vi "hmi_peg_leg.vi"(11 "UserData":T1) -> ()   [LabVIEW 2011]
uses:
  user_data.ctl
  user_buttons_dualaction.ctl
  user_buttons_360.ctl
  joe_johnson/peg_leg_state.ctl
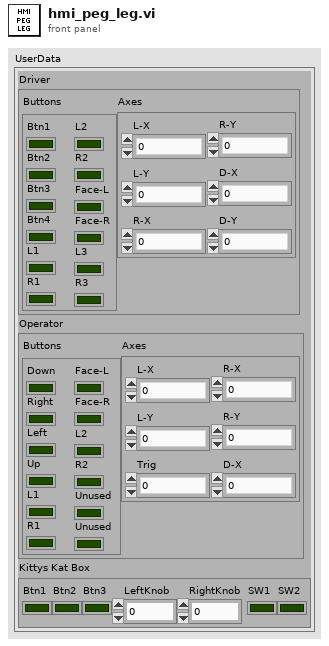
[diagram p1: front panel]
types:
  T1 = typedef "user_data.ctl" = cluster{"Driver":cluster{"Buttons":T2, "Axes":cluster{"L-X":dbl, "L-Y":dbl, "R-X":dbl, "R-Y":dbl, "D-X":dbl, "D-Y":dbl}}, "Operator":cluster{"Buttons":T3, "Axes":cluster{"L-X":dbl, "L-Y":dbl, "Trig":dbl, "R-X":dbl, "R-Y":dbl, "D-X":dbl}}, "Kittys Kat Box":cluster{"Btn1":bool, "Btn2":bool, "Btn3":bool, "LeftKnob":dbl, "RightKnob":dbl, "SW1":bool, "SW2":bool}}
  T2 = typedef "user_buttons_dualaction.ctl" = cluster{"Btn1":bool, "Btn2":bool, "Btn3":bool, "Btn4":bool, "L1":bool, "R1":bool, "L2":bool, "R2":bool, "Face-L":bool, "Face-R":bool, "L3":bool, "R3":bool}
  T3 = typedef "user_buttons_360.ctl" = cluster{"Down":bool, "Right":bool, "Left":bool, "Up":bool, "L1":bool, "R1":bool, "Face-L":bool, "Face-R":bool, "L2":bool, "R2":bool, "Unused":bool, "Unused":bool}
  T4 = typedef "peg_leg_state.ctl" = enum16{"up", "down", "unfold", "manual"}
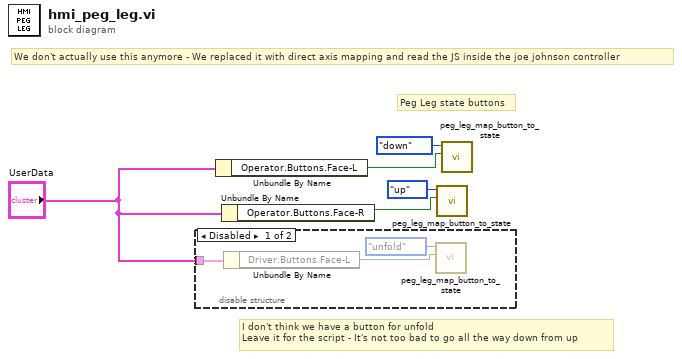
[diagram p0: block diagram]
diagram:
  # "We don't actually use this anymore - We replaced it with direct axis mapping and read the JS inside the joe johnson controller"
  # "I don't think we have a button for unfold\nLeave it for the script - It's not too bad to go all the way down from up"
  # "Peg Leg state buttons"
  n1 = disable-structure shown="Disabled" {
    disable-tunnel: "UserData" -> [w7 _]
    frame Disabled {
      n2 = Unbundle By Name(w7) -> ("Driver.Buttons.Face-L"=w6:bool)
      n3 = call "peg_leg_map_button_to_state.vi"("Button"=w6, "peg_leg_state"=peg_leg_state."unfold") -> ()  [unwired: 10 in]
    }
    frame Enabled {
    }
  }
  n4 = Unbundle By Name("UserData") -> ("Operator.Buttons.Face-L"=w4:bool)
  n5 = Unbundle By Name("UserData") -> ("Operator.Buttons.Face-R"=w5:bool)
  n6 = call "peg_leg_map_button_to_state.vi"("Button"=w5, "peg_leg_state"=peg_leg_state."up") -> ()  [unwired: 10 in]
  n7 = call "peg_leg_map_button_to_state.vi"("Button"=w4, "peg_leg_state"=peg_leg_state."down") -> ()  [unwired: 10 in]
